vi "getValFromVariant.vi"   [LabVIEW 2018]
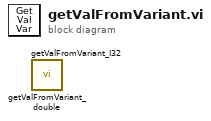
[diagram p0: block diagram]
diagram:
  n1 = call "getValFromVariant_double.vi"() -> ()  [unwired: 10 in, 2 out]
  n2 = call "getValFromVariant_I32.vi"() -> ()  [unwired: 10 in, 2 out]
